vi "Write Max.vi"(8 "error in (no error)":errorcluster, 10 "Max":dbl, 11 "IV_meas in":refnum<class "IV_meas.lvclass">) -> (0 "error out":errorcluster, 3 "IV_meas out":refnum<class "IV_meas.lvclass">)   [LabVIEW 2014, in "IV_meas.lvclass"]
uses:
  IV_meas.lvclass
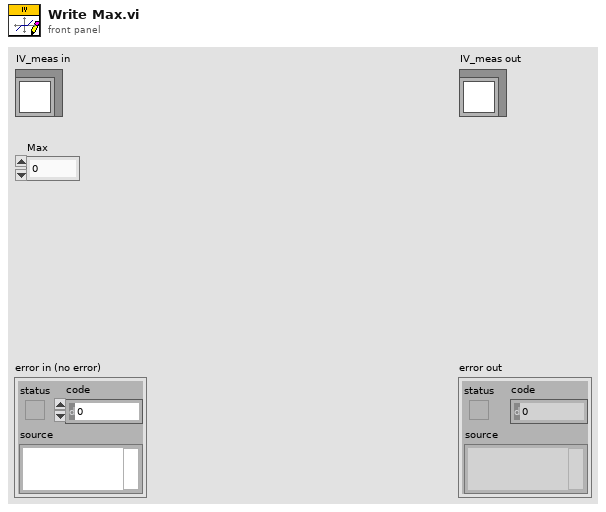
[diagram p1: front panel]
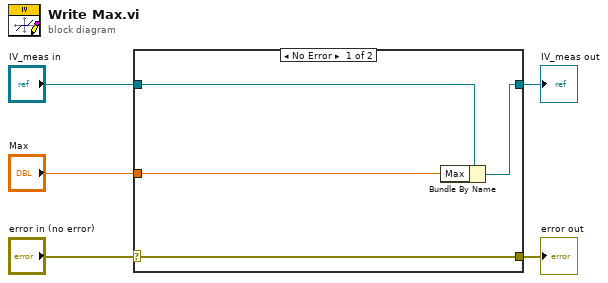
[diagram p0: block diagram]
diagram:
  n1 = case shown="No Error" "error in (no error)" {
    selector: "error in (no error)" -> [w9 w10]
    tunnel: [w9 w10] -> w4
    tunnel: [w7 w11] -> w2
    tunnel: "IV_meas in" -> [w8 w11]
    tunnel: "Max" -> [w6 _]
    frame No Error {
      n2 = Bundle By Name(cluster=w8, "Max"=w6) -> (w7:refnum<class "IV_meas.lvclass">)
    }
    frame Error {
    }
  }
  "error out" <- w4
  "IV_meas out" <- w2
